vi "Determine Transmit.vi"(7 "Current Time":u32, 9 "Detect?":bool[](array[boolean]), 10 "Values":dbl[](array[numeric]), 11 "Frame Settings in":T1 {"Protection Configurations"."CRC Channels"."Data Type" items=["Signed", "Unsigned", "IEEE Float"]}) -> (1 "Transmit":bool, 2 "Values out":dbl[](array[numeric]), 3 "Frame Settings out":T1 {"Protection Configurations"."CRC Channels"."Data Type" items=["Signed", "Unsigned", "IEEE Float"]})   [LabVIEW 2024, in "Protection and Counter Support Engine.lvlib"]
uses:
  Protection and Counter Support Engine.lvlib
  Types/RT Frame Settings.ctl
  Shared/Types/Exported Frame Type.ctl
  Types/RT Protection Configuration.ctl
  Shared/Types/Protection Type.ctl
  Shared/Types/XNET Signal Configuration.ctl
  Shared/Types/Exported Counter Settings.ctl
  Shared/Types/Exported Event Trigger Type.ctl
  Shared/Protection and Counter Support Shared.lvlib
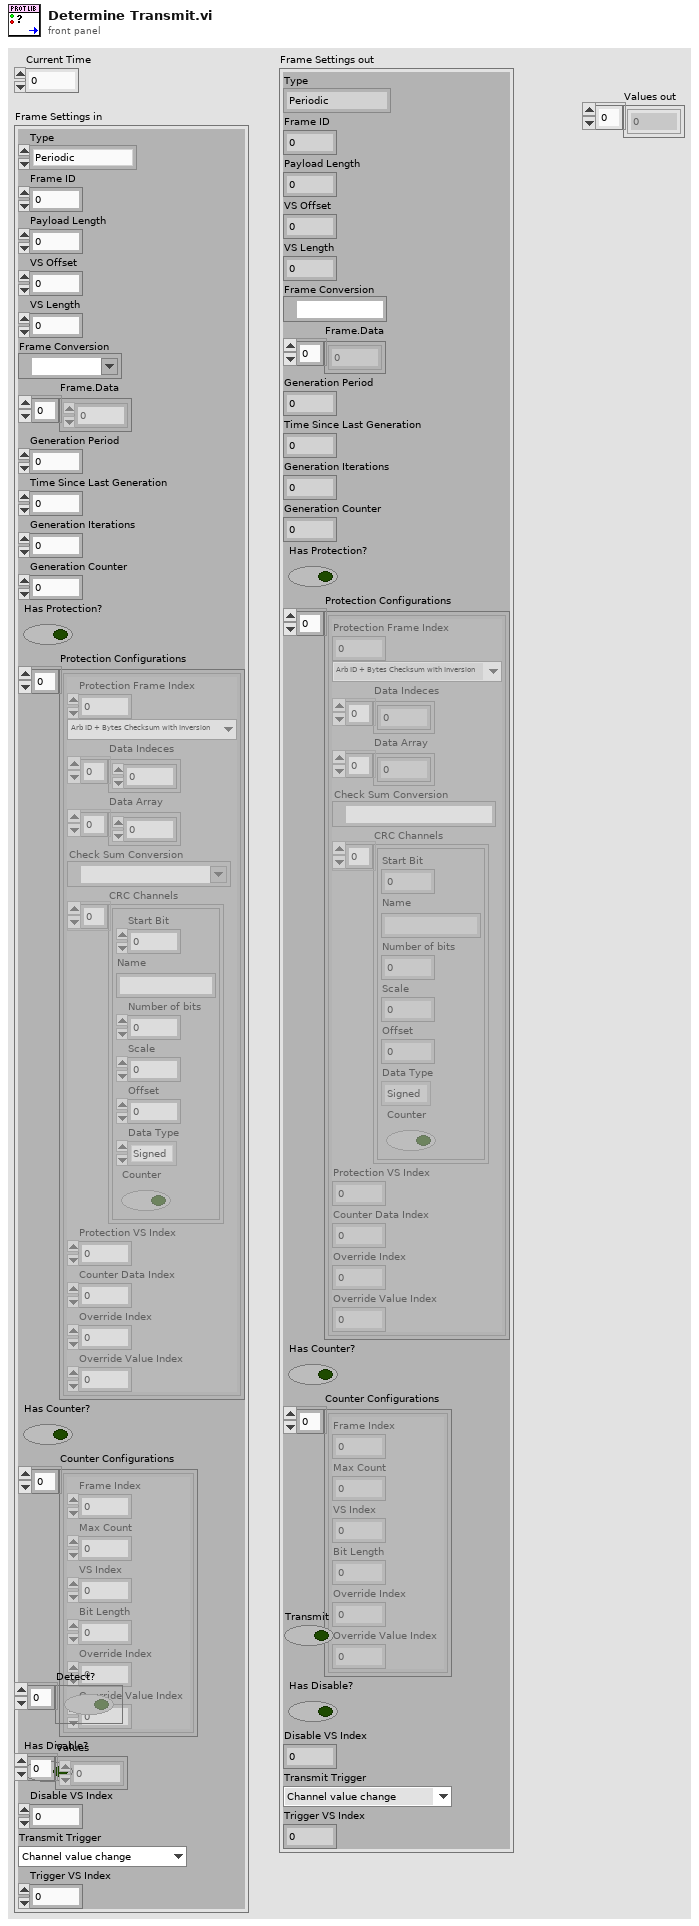
[diagram p1: front panel]
types:
  T1 = typedef "Protection and Counter Support Engine.lvlib/RT Frame Settings.ctl" = cluster{"Type":T2, "Frame ID":u32, "Payload Length":u32, "VS Offset":i32, "VS Length":i32, "Frame Conversion":refnum<k21>, "Frame.Data":dbl[], "Generation Period":u32, "Time Since Last Generation":u32, "Generation Iterations":u32, "Generation Counter":u32, "Has Protection?":bool, "Protection Configurations":T3[], "Has Counter?":bool, "Counter Configurations":T6[], "Has Disable?":bool, "Disable VS Index":i32, "Transmit Trigger":T7, "Trigger VS Index":i32}
  T2 = typedef "Protection and Counter Support Shared.lvlib/Exported Frame Type.ctl" = enum16{"Periodic", "Event", "Periodic/Event"}
  T3 = typedef "Protection and Counter Support Engine.lvlib/RT Protection Configuration.ctl" = cluster{"Protection Frame Index":i32, "Protection Type":T4, "Data Indeces":i32[], "Data Array":dbl[], "Check Sum Conversion":refnum<k21>, "CRC Channels":T5[], "Protection VS Index":i32, "Counter Data Index":i32, "Override Index":i32, "Override Value Index":i32}
  T4 = typedef "Protection and Counter Support Shared.lvlib/Protection Type.ctl" = enum16{"Arb ID + Bytes Checksum with Inversion", "Arb ID + Bytes CRC with Inversion", "Reversed Raw Signal Checksum with Inversion", "Concatenated Two's Compliment"}
  T5 = typedef "Protection and Counter Support Shared.lvlib/XNET Signal Configuration.ctl" = cluster{"Start Bit":i32, "Name":string, "Number of bits":i32, "Scale":dbl, "Offset":dbl, "Data Type":u32, "Counter":bool}
  T6 = typedef "Protection and Counter Support Shared.lvlib/Exported Counter Settings.ctl" = cluster{"Frame Index":i32, "Max Count":dbl, "VS Index":i32, "Bit Length":i64, "Override Index":i32, "Override Value Index":i32}
  T7 = typedef "Protection and Counter Support Shared.lvlib/Exported Event Trigger Type.ctl" = enum16{"Channel value change", "Trigger channel (not zero)", "Channel value change or trigger channel (not zero)", "Trigger channel (any value change)", "Channel value change or trigger channel (any value change)"}
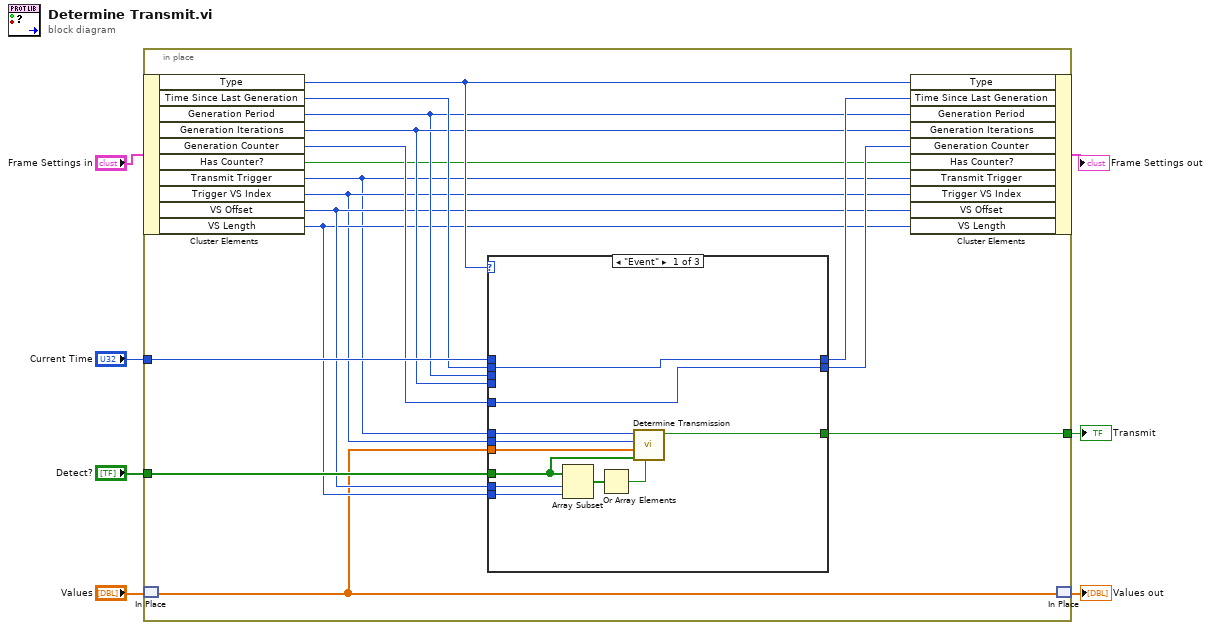
[diagram p0: block diagram]
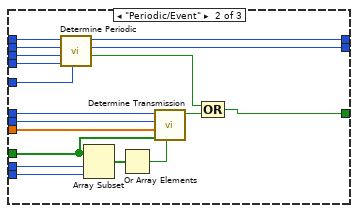
[diagram p2: hidden frame]
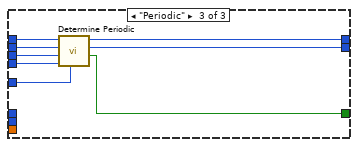
[diagram p3: hidden frame]
diagram:
  n1 = in-place {
    in-place-border: [w23] -> w7
    in-place-border: "Detect?" -> [w22]
    in-place-border: "Current Time" -> [w21]
    n2 = in-place-cluster #1("Frame Settings in") -> ("Type"=w18:T2, "Time Since Last Generation"=w19:u32, "Generation Period"=w14:u32, "Generation Iterations"=w15:u32, "Generation Counter"=w20:u32, "Has Counter?"=w13:bool, "Transmit Trigger"=w9:T7, "Trigger VS Index"=w10:i32, "VS Offset"=w12:i32, "VS Length"=w11:i32)
    n3 = in-place-match #2("Values") -> (w8:dbl[])
    n4 = case shown="\"Event\"" w18 {
      tunnel: w14 -> [_ w42 w60]
      tunnel: w19 -> [w34 w41 w59]
      tunnel: w21 -> [_ w40 w58]
      tunnel: [w34 w39 w57] -> w17
      tunnel: w20 -> [w33 w44 w53]
      tunnel: w15 -> [_ w43 w54]
      tunnel: [w26 w35 w56] -> w23
      tunnel: [w33 w38 w55] -> w16
      tunnel: w9 -> [w28 w48 _]
      tunnel: w10 -> [w29 w49 _]
      tunnel: w11 -> [w32 w52 _]
      tunnel: w12 -> [w31 w51 _]
      tunnel: w22 -> [w25 w46 _]
      tunnel: w8 -> [w24 w45 _]
      frame "Event" {
        n5 = Array Subset(array=w25, index=w31, length=w32) -> (w30:bool[])
        n6 = Or Array Elements(Boolean array=w30) -> (logical OR=w27:bool)
        n7 = call "Determine Transmission.vi"("Channel Value Change"=w27, "Detect?"=w25, "Values"=w24, "Trigger VS Index"=w29, "Transmit Trigger"=w28) -> ("Transmit"=w26:bool)  [unwired: 6 in]
      }
      frame "Periodic/Event" {
        n8 = call "Determine Periodic.vi"("Generation Counter"=w44, "Generation Iterations"=w43, "Generation Period"=w42, "Time Since Last Generation in"=w41, "Current Time"=w40) -> ("Tranmit"=w37:bool, "Generation Counter out"=w38:u32, "Time Since Last Generation out"=w39:u32)  [unwired: 4 in]
        n9 = Array Subset(array=w46, index=w51, length=w52) -> (w50:bool[])
        n10 = Or Array Elements(Boolean array=w50) -> (logical OR=w47:bool)
        n11 = call "Determine Transmission.vi"("Channel Value Change"=w47, "Detect?"=w46, "Values"=w45, "Trigger VS Index"=w49, "Transmit Trigger"=w48) -> ("Transmit"=w36:bool)  [unwired: 6 in]
        n12 = Compound Arithmetic op=OR(w37, w36) -> (w35:bool)
      }
      frame "Periodic" {
        n13 = call "Determine Periodic.vi"("Generation Counter"=w53, "Generation Iterations"=w54, "Generation Period"=w60, "Time Since Last Generation in"=w59, "Current Time"=w58) -> ("Tranmit"=w56:bool, "Generation Counter out"=w55:u32, "Time Since Last Generation out"=w57:u32)  [unwired: 4 in]
      }
    }
    n14 = in-place-cluster #1("Type"=w18, "Time Since Last Generation"=w17, "Generation Period"=w14, "Generation Iterations"=w15, "Generation Counter"=w16, "Has Counter?"=w13, "Transmit Trigger"=w9, "Trigger VS Index"=w10, "VS Offset"=w12, "VS Length"=w11) -> (→"Frame Settings out":T1)
    n15 = in-place-match #2(w8) -> (→"Values out":dbl[])
  }
  "Transmit" <- w7
